vi "writeToXML.vi"(8 "error in (no error)":errorcluster, 10 "ClassLabel":string, 11 "FocusSelect in":refnum<class "FocusSelect.lvclass">) -> (0 "error out":errorcluster, 2 "XML out":string, 3 "FocusSelect out":refnum<class "FocusSelect.lvclass">)   [LabVIEW 2014, in "TCSDataDefinitions.lvlib" / "TCSCommand.lvlib" / "FocusSelect.lvclass"]
uses:
  FocusSelect.lvclass
  FocusSelect.lvclass/FocusSelect.ctl
  TCSTcsCommand/TCSTcsCommand.lvclass
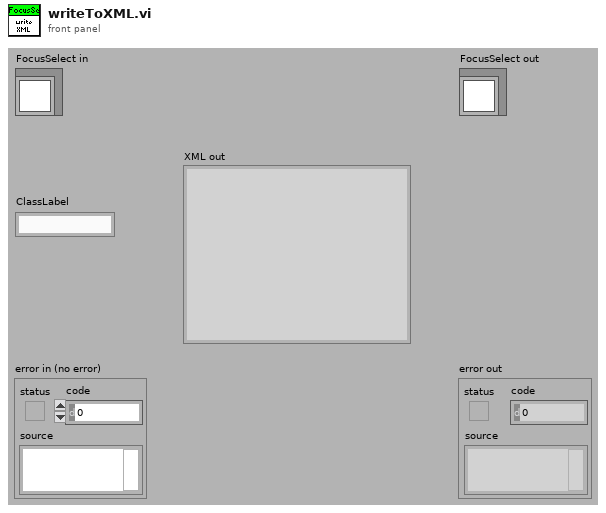
[diagram p1: front panel]
types:
  T1 = typedef "TCSDataDefinitions.lvlib/TCSCommand.lvlib/FocusNameTypes.ctl" = enum16{"Cass", "Prime", "Nasmyth1", "Nasmyth2", "BentCass1", "BentCass2", "BentCass3", "BentCass4", "BentCass5", "BentCass6"}
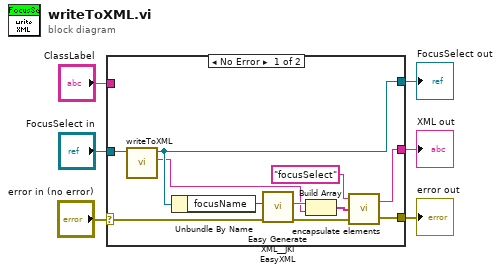
[diagram p0: block diagram]
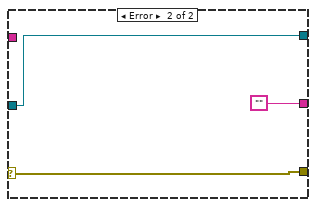
[diagram p2: hidden frame]
diagram:
  n1 = case shown="No Error" "error in (no error)" {
    selector: "error in (no error)" -> [w13 w20]
    tunnel: [w12 w20] -> w5
    tunnel: [w9 w19] -> w3
    tunnel: "FocusSelect in" -> [w10 w19]
    tunnel: "ClassLabel" -> [_ _]
    tunnel: [w11 ""] -> w1
    frame No Error {
      n2 = call-parent "writeToXML.vi"("TCSTcsCommand in"=w10) -> ("XML out"=w8:string, "TCSTcsCommand out"=w9:refnum<class "FocusSelect.lvclass">)  [unwired: 8 in, 1 out]
      n3 = Unbundle By Name(w9) -> ("focusName"=w17:T1)
      n4 = call <vilib>:"Easy Generate XML__JKI EasyXML.vi"("error in (no error)"=w13, "LabVIEW Data"=w17) -> ("error out"=w14:errorcluster, "XML String"=w16:string)  [unwired: 8 in]
      n5 = Build Array(w16, w8) -> (w15:string[])
      n6 = call "encapsulate elements.vi"("error in"=w14, "Elements"=w15, "Class Label"="focusSelect") -> ("error out"=w12:errorcluster, "XML out"=w11:string)
    }
    frame Error {
    }
  }
  "error out" <- w5
  "FocusSelect out" <- w3
  "XML out" <- w1
